vi "Card PXI Information.vi"() -> ()   [LabVIEW 2019]
doc: "This example reports the card PXI signal information, displays the current state\nof the various PXI discrete I/O pins, is capable of configuring PXI discrete I/Os as \noutput using the \"Enable\" toggle, Assert or Deassert output-enabled signals using \nthe \"Drive\" toggle and is capable of sourcing the 10MHz timing signal on the \nDSTARC line."
uses:
  <instrlib>/BTICardLib/Public/Controls/PXI Signal.ctl
  <instrlib>/BTICardLib/Private/Initialize By Card Number and Core Number.vi
  <instrlib>/BTICardLib/BTICardLV.lvlib
panel:
  out "?":bool
  out "?":bool
  out "?":bool
  out "?":bool
  out "?":bool
  out "?":bool
  out "?":bool
  out "?":bool
  out "?":bool
  out "?":bool
  out "?":bool
  in  "?":bool
  in  "?":bool
  in  "?":bool
  in  "?":bool
  in  "?":bool
  in  "?":bool
  in  "?":bool
  in  "?":bool
  in  "?":bool
  in  "?":bool
  in  "?":bool
  in  "?":bool
  in  "?":bool
  in  "?":bool
  in  "?":bool
  in  "?":bool
  in  "?":bool
  in  "?":bool
  in  "?":bool
  in  "?":bool
  in  "?":bool
  in  "?":bool
  in  "?":bool
  in  "?":bool
  in  "?":bool
  out "?":bool
  in  "Card Number":i32
  in  "Core Number":i32
  # "Card PXI Information"
  # "©2016 Astronics Ballard Technology"
  # "This example reports the card PXI signal information, displays the current state\nof the various PXI discrete I/O pins, is capable of configuring PXI discrete I/Os as \noutput using the \"Enable\" toggle, Assert or Deassert output-enabled signals using \nthe \"Drive\" toggle and is capable of sourcing the 10MHz timing signal on the \nDSTARC line."
  # "Signal High/Low"
  # "Enable"
  # "Drive"
  # "PXI_TRIG0"
  # "PXI_TRIG1"
  # "PXI_TRIG2"
  # "PXI_TRIG3"
  # "PXI_TRIG4"
  # "PXI_TRIG5"
  # "PXI_TRIG6"
  # "PXI_TRIG7"
  # "PXIE_DSTARA"
  # "PXIE_DSTARB"
  # "PXI_STAR"
  # "PXIE_DSTARC"
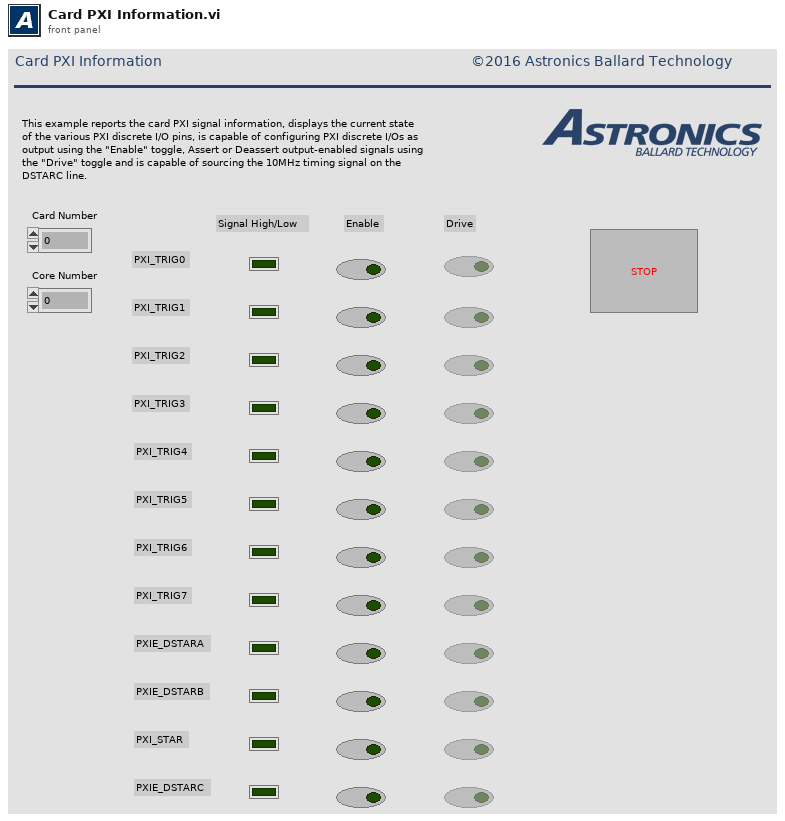
[diagram p1: front panel]
types:
  T1 = enum8{"Enabled", "Disabled", "Disabled and Grayed Out"}
  T2 = typedef "BTICardLV.lvlib/PXI Signal.ctl" = u32
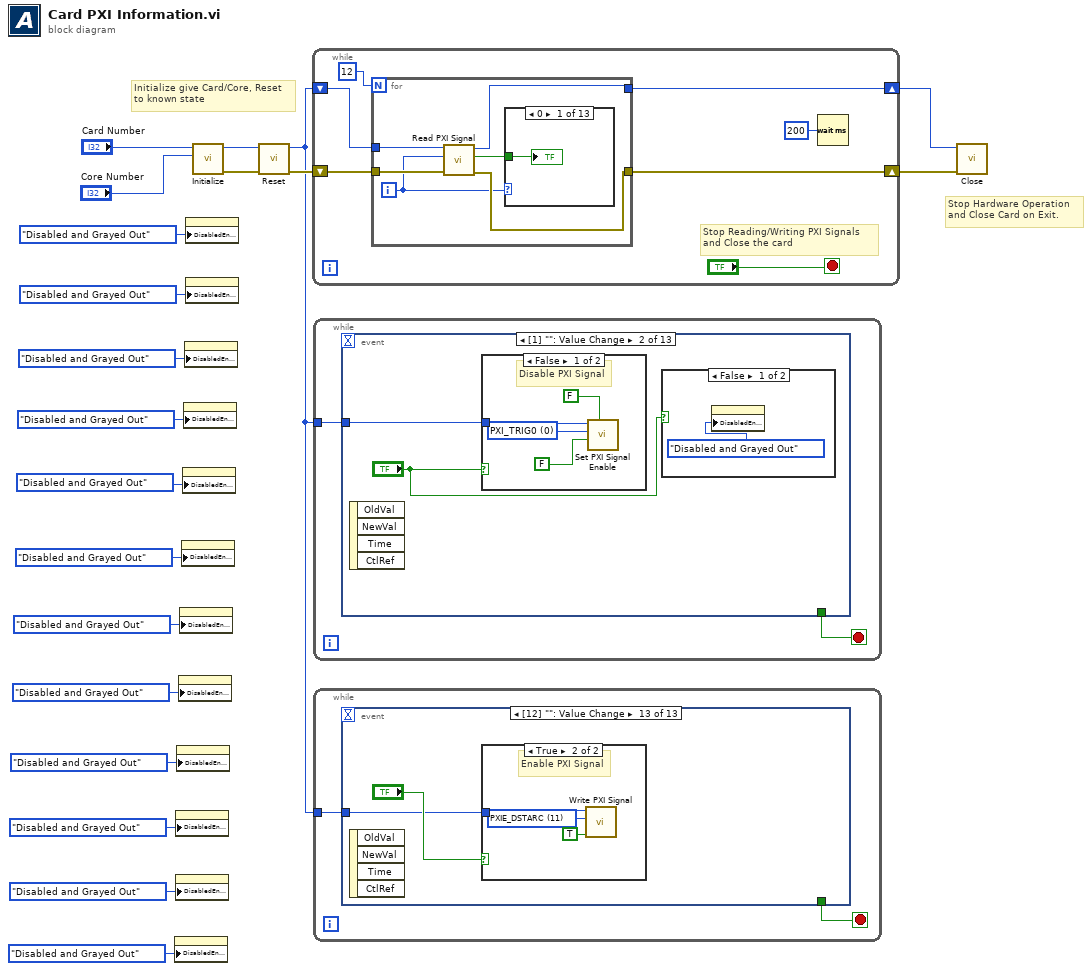
[diagram p0: block diagram]
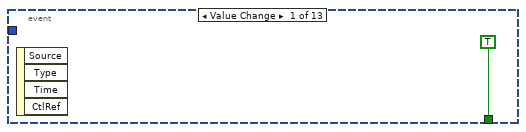
[diagram p2: hidden frame]
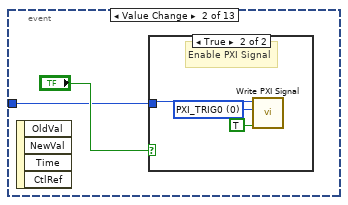
[diagram p3: hidden frame]
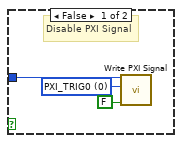
[diagram p4: hidden frame]
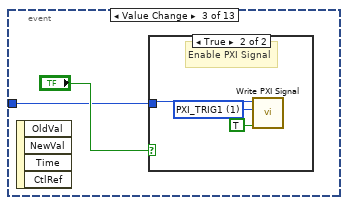
[diagram p5: hidden frame]
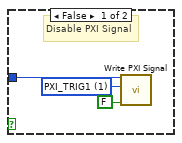
[diagram p6: hidden frame]
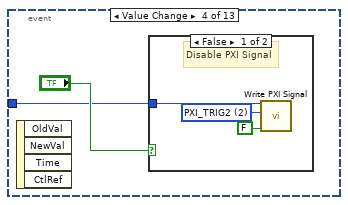
[diagram p7: hidden frame]
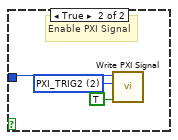
[diagram p8: hidden frame]
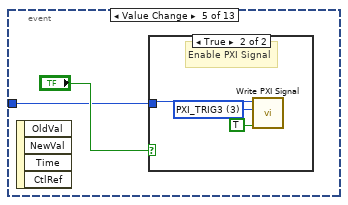
[diagram p9: hidden frame]
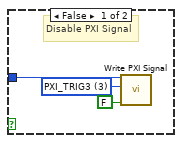
[diagram p10: hidden frame]
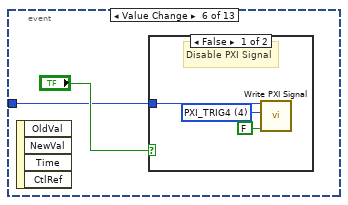
[diagram p11: hidden frame]
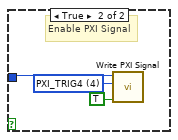
[diagram p12: hidden frame]
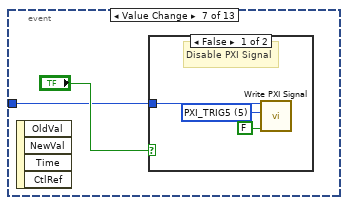
[diagram p13: hidden frame]
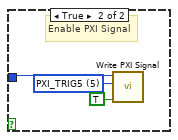
[diagram p14: hidden frame]
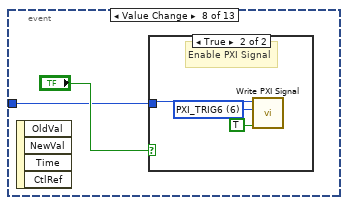
[diagram p15: hidden frame]
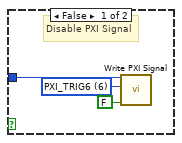
[diagram p16: hidden frame]
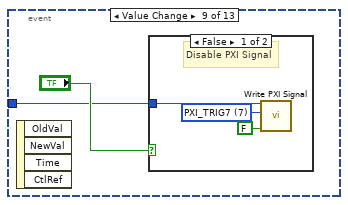
[diagram p17: hidden frame]
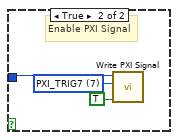
[diagram p18: hidden frame]
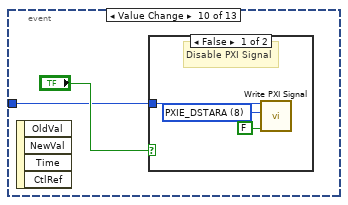
[diagram p19: hidden frame]
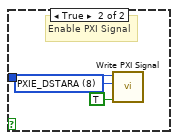
[diagram p20: hidden frame]
diagram:
  # "Stop Hardware Operation\nand Close Card on Exit."
  # "Initialize give Card/Core, Reset\nto known state"
  n1 = property class="Bool (strict)"("DisabledEnum"=T1."Disabled and Grayed Out" ("Disabled")) -> ()  [unwired: 2 in, 2 out]
  n2 = property class="Bool (strict)"("DisabledEnum"=T1."Disabled and Grayed Out" ("Disabled")) -> ()  [unwired: 2 in, 2 out]
  n3 = property class="Bool (strict)"("DisabledEnum"=T1."Disabled and Grayed Out" ("Disabled")) -> ()  [unwired: 2 in, 2 out]
  n4 = property class="Bool (strict)"("DisabledEnum"=T1."Disabled and Grayed Out" ("Disabled")) -> ()  [unwired: 2 in, 2 out]
  n5 = property class="Bool (strict)"("DisabledEnum"=T1."Disabled and Grayed Out" ("Disabled")) -> ()  [unwired: 2 in, 2 out]
  n6 = property class="Bool (strict)"("DisabledEnum"=T1."Disabled and Grayed Out" ("Disabled")) -> ()  [unwired: 2 in, 2 out]
  n7 = property class="Bool (strict)"("DisabledEnum"=T1."Disabled and Grayed Out" ("Disabled")) -> ()  [unwired: 2 in, 2 out]
  n8 = property class="Bool (strict)"("DisabledEnum"=T1."Disabled and Grayed Out" ("Disabled")) -> ()  [unwired: 2 in, 2 out]
  n9 = property class="Bool (strict)"("DisabledEnum"=T1."Disabled and Grayed Out" ("Disabled")) -> ()  [unwired: 2 in, 2 out]
  n10 = property class="Bool (strict)"("DisabledEnum"=T1."Disabled and Grayed Out" ("Disabled")) -> ()  [unwired: 2 in, 2 out]
  n11 = property class="Bool (strict)"("DisabledEnum"=T1."Disabled and Grayed Out" ("Disabled")) -> ()  [unwired: 2 in, 2 out]
  n12 = property class="Bool (strict)"("DisabledEnum"=T1."Disabled and Grayed Out" ("Disabled")) -> ()  [unwired: 2 in, 2 out]
  n13 = call-poly <instrlib>:"Initialize.vi"("core number"="Core Number", "card number"="Card Number") -> ("error out"=w17:errorcluster, "core handle out"=w18:u64)  [unwired: 8 in]
  n14 = call <instrlib>:"Reset.vi"("error in (no error)"=w17, "core handle in"=w18) -> ("error out"=w16:errorcluster, "core handle out"=w13:u64)  [unwired: 8 in]
  n15 = while {
    shift-right: [w23] -> w14
    shift-left: w13 -> [w26]
    shift-right: [w24] -> w15
    shift-left: w16 -> [w25]
    stop <- "?" stop-if-true
    # "Stop Reading/Writing PXI Signals\nand Close the card"
    n16 = for {
      N: 12 -> [_]
      tunnel: w26 -> [w33]
      tunnel: w25 -> [w32]
      tunnel: [w31] -> w24
      tunnel: [w30] -> w23
      i -> [w29]
      n17 = call <instrlib>:"Read PXI Signal.vi"("error in (no error)"=w32, "pxi signal"=w29, "core handle in"=w33) -> ("error out"=w31:errorcluster, "signal value"=w28:bool, "core handle out"=w30:u64)  [unwired: 6 in]
      n18 = case shown="0" w29 {
        tunnel: w28 -> [w34 w35 w36 w37 w38 w39 w40 w41 w42 w43 w44 w45 _]
        frame 0 {
          "?" <- w34
        }
        frame 1 {
          "?" <- w35
        }
        frame 2 {
          "?" <- w36
        }
        frame 3 {
          "?" <- w37
        }
        frame 4 {
          "?" <- w38
        }
        frame 5 {
          "?" <- w39
        }
        frame 6 {
          "?" <- w40
        }
        frame 7 {
          "?" <- w41
        }
        frame 8 {
          "?" <- w42
        }
        frame 9 {
          "?" <- w43
        }
        frame 10 {
          "?" <- w44
        }
        frame 11 {
          "?" <- w45
        }
        frame 12, Default {
        }
      }
    }
    n19 = Wait (ms)(milliseconds to wait=u32 200) -> ()  [unwired: 1 out]
  }
  n20 = while {
    tunnel: w13 -> [w47]
    stop <- w46 stop-if-true
    n21 = event shown="[1] \"\": Value Change" {
      selector: _ -> [_ _ _ _ _ _ _ _ _ _ _ _ _]
      dyn-events: _ -> [_ _ _ _ _ _ _ _ _ _ _ _ _]
      timeout: _ -> [_ _ _ _ _ _ _ _ _ _ _ _ _]
      tunnel: w47 -> [_ w49 w61 w73 w85 w97 w109 w121 w133 w145 w157 w169 w181]
      tunnel: [TRUE ("Stop Reading/Writing PXI Signals\nand Close the card") _ _ _ _ _ _ _ _ _ _ _ _] -> w46
      event Value Change {
        n22 = event-data() -> ()  [unwired: 1 in, 4 out]
      }
      event Value Change {
        n23 = event-data() -> ()  [unwired: 1 in, 4 out]
        n24 = case shown="False" "?" {
          tunnel: w49 -> [w54 w60]
          frame False {
            w55 = T2 0 items=["PXI_TRIG0", "PXI_TRIG1", "PXI_TRIG2", "PXI_TRIG3", "PXI_TRIG4", "PXI_TRIG5", "PXI_TRIG6", "PXI_TRIG7", "PXIE_DSTARA", "PXIE_DSTARB", "PXI_STAR", "PXIE_DSTARC"] ("pxi signal")
            # "Disable PXI Signal"
            n25 = call <instrlib>:"Set PXI Signal Enable.vi"("signal value"=FALSE, "output enable?"=FALSE, "pxi signal"=w55, "corehandle in"=w54) -> ()  [unwired: 6 in, 2 out]
          }
          frame True {
            w58 = T2 0 items=["PXI_TRIG0", "PXI_TRIG1", "PXI_TRIG2", "PXI_TRIG3", "PXI_TRIG4", "PXI_TRIG5", "PXI_TRIG6", "PXI_TRIG7", "PXIE_DSTARA", "PXIE_DSTARB", "PXI_STAR", "PXIE_DSTARC"] ("pxi signal")
            # "Enable PXI Signal"
            n26 = call <instrlib>:"Set PXI Signal Enable.vi"("signal value"=FALSE, "output enable?"=TRUE, "pxi signal"=w58, "corehandle in"=w60) -> ()  [unwired: 6 in, 2 out]
          }
        }
        n27 = case shown="False" "?" {
          frame False {
            n28 = property class="Bool (strict)"("DisabledEnum"=T1."Disabled and Grayed Out" ("Disabled")) -> ()  [unwired: 2 in, 2 out]
          }
          frame True {
            n29 = property class="Bool (strict)"("DisabledEnum"=T1."Enabled" ("Disabled")) -> ()  [unwired: 2 in, 2 out]
          }
        }
      }
      event Value Change {
        n30 = event-data() -> ()  [unwired: 1 in, 4 out]
        n31 = case shown="True" "?" {
          tunnel: w61 -> [w66 w72]
          frame False {
            w67 = T2 1 items=["PXI_TRIG0", "PXI_TRIG1", "PXI_TRIG2", "PXI_TRIG3", "PXI_TRIG4", "PXI_TRIG5", "PXI_TRIG6", "PXI_TRIG7", "PXIE_DSTARA", "PXIE_DSTARB", "PXI_STAR", "PXIE_DSTARC"] ("pxi signal")
            # "Disable PXI Signal"
            n32 = call <instrlib>:"Set PXI Signal Enable.vi"("signal value"=FALSE, "output enable?"=FALSE, "pxi signal"=w67, "corehandle in"=w66) -> ()  [unwired: 6 in, 2 out]
          }
          frame True {
            w70 = T2 1 items=["PXI_TRIG0", "PXI_TRIG1", "PXI_TRIG2", "PXI_TRIG3", "PXI_TRIG4", "PXI_TRIG5", "PXI_TRIG6", "PXI_TRIG7", "PXIE_DSTARA", "PXIE_DSTARB", "PXI_STAR", "PXIE_DSTARC"] ("pxi signal")
            # "Enable PXI Signal"
            n33 = call <instrlib>:"Set PXI Signal Enable.vi"("signal value"=FALSE, "output enable?"=TRUE, "pxi signal"=w70, "corehandle in"=w72) -> ()  [unwired: 6 in, 2 out]
          }
        }
        n34 = case shown="True" "?" {
          frame False {
            n35 = property class="Bool (strict)"("DisabledEnum"=T1."Disabled and Grayed Out" ("Disabled")) -> ()  [unwired: 2 in, 2 out]
          }
          frame True {
            n36 = property class="Bool (strict)"("DisabledEnum"=T1."Enabled" ("Disabled")) -> ()  [unwired: 2 in, 2 out]
          }
        }
      }
      event Value Change {
        n37 = event-data() -> ()  [unwired: 1 in, 4 out]
        n38 = case shown="True" "?" {
          tunnel: w73 -> [w78 w84]
          frame False {
            w79 = T2 2 items=["PXI_TRIG0", "PXI_TRIG1", "PXI_TRIG2", "PXI_TRIG3", "PXI_TRIG4", "PXI_TRIG5", "PXI_TRIG6", "PXI_TRIG7", "PXIE_DSTARA", "PXIE_DSTARB", "PXI_STAR", "PXIE_DSTARC"] ("pxi signal")
            # "Disable PXI Signal"
            n39 = call <instrlib>:"Set PXI Signal Enable.vi"("signal value"=FALSE, "output enable?"=FALSE, "pxi signal"=w79, "corehandle in"=w78) -> ()  [unwired: 6 in, 2 out]
          }
          frame True {
            w82 = T2 2 items=["PXI_TRIG0", "PXI_TRIG1", "PXI_TRIG2", "PXI_TRIG3", "PXI_TRIG4", "PXI_TRIG5", "PXI_TRIG6", "PXI_TRIG7", "PXIE_DSTARA", "PXIE_DSTARB", "PXI_STAR", "PXIE_DSTARC"] ("pxi signal")
            # "Enable PXI Signal"
            n40 = call <instrlib>:"Set PXI Signal Enable.vi"("signal value"=FALSE, "output enable?"=TRUE, "pxi signal"=w82, "corehandle in"=w84) -> ()  [unwired: 6 in, 2 out]
          }
        }
        n41 = case shown="True" "?" {
          frame False {
            n42 = property class="Bool (strict)"("DisabledEnum"=T1."Disabled and Grayed Out" ("Disabled")) -> ()  [unwired: 2 in, 2 out]
          }
          frame True {
            n43 = property class="Bool (strict)"("DisabledEnum"=T1."Enabled" ("Disabled")) -> ()  [unwired: 2 in, 2 out]
          }
        }
      }
      event Value Change {
        n44 = event-data() -> ()  [unwired: 1 in, 4 out]
        n45 = case shown="False" "?" {
          tunnel: w85 -> [w90 w96]
          frame False {
            w91 = T2 3 items=["PXI_TRIG0", "PXI_TRIG1", "PXI_TRIG2", "PXI_TRIG3", "PXI_TRIG4", "PXI_TRIG5", "PXI_TRIG6", "PXI_TRIG7", "PXIE_DSTARA", "PXIE_DSTARB", "PXI_STAR", "PXIE_DSTARC"] ("pxi signal")
            # "Disable PXI Signal"
            n46 = call <instrlib>:"Set PXI Signal Enable.vi"("signal value"=FALSE, "output enable?"=FALSE, "pxi signal"=w91, "corehandle in"=w90) -> ()  [unwired: 6 in, 2 out]
          }
          frame True {
            w94 = T2 3 items=["PXI_TRIG0", "PXI_TRIG1", "PXI_TRIG2", "PXI_TRIG3", "PXI_TRIG4", "PXI_TRIG5", "PXI_TRIG6", "PXI_TRIG7", "PXIE_DSTARA", "PXIE_DSTARB", "PXI_STAR", "PXIE_DSTARC"] ("pxi signal")
            # "Enable PXI Signal"
            n47 = call <instrlib>:"Set PXI Signal Enable.vi"("signal value"=FALSE, "output enable?"=TRUE, "pxi signal"=w94, "corehandle in"=w96) -> ()  [unwired: 6 in, 2 out]
          }
        }
        n48 = case shown="False" "?" {
          frame False {
            n49 = property class="Bool (strict)"("DisabledEnum"=T1."Disabled and Grayed Out" ("Disabled")) -> ()  [unwired: 2 in, 2 out]
          }
          frame True {
            n50 = property class="Bool (strict)"("DisabledEnum"=T1."Enabled" ("Disabled")) -> ()  [unwired: 2 in, 2 out]
          }
        }
      }
      event Value Change {
        n51 = event-data() -> ()  [unwired: 1 in, 4 out]
        n52 = case shown="True" "?" {
          tunnel: w97 -> [w102 w108]
          frame False {
            w103 = T2 4 items=["PXI_TRIG0", "PXI_TRIG1", "PXI_TRIG2", "PXI_TRIG3", "PXI_TRIG4", "PXI_TRIG5", "PXI_TRIG6", "PXI_TRIG7", "PXIE_DSTARA", "PXIE_DSTARB", "PXI_STAR", "PXIE_DSTARC"] ("pxi signal")
            # "Disable PXI Signal"
            n53 = call <instrlib>:"Set PXI Signal Enable.vi"("signal value"=FALSE, "output enable?"=FALSE, "pxi signal"=w103, "corehandle in"=w102) -> ()  [unwired: 6 in, 2 out]
          }
          frame True {
            w106 = T2 4 items=["PXI_TRIG0", "PXI_TRIG1", "PXI_TRIG2", "PXI_TRIG3", "PXI_TRIG4", "PXI_TRIG5", "PXI_TRIG6", "PXI_TRIG7", "PXIE_DSTARA", "PXIE_DSTARB", "PXI_STAR", "PXIE_DSTARC"] ("pxi signal")
            # "Enable PXI Signal"
            n54 = call <instrlib>:"Set PXI Signal Enable.vi"("signal value"=FALSE, "output enable?"=TRUE, "pxi signal"=w106, "corehandle in"=w108) -> ()  [unwired: 6 in, 2 out]
          }
        }
        n55 = case shown="True" "?" {
          frame False {
            n56 = property class="Bool (strict)"("DisabledEnum"=T1."Disabled and Grayed Out" ("Disabled")) -> ()  [unwired: 2 in, 2 out]
          }
          frame True {
            n57 = property class="Bool (strict)"("DisabledEnum"=T1."Enabled" ("Disabled")) -> ()  [unwired: 2 in, 2 out]
          }
        }
      }
      event Value Change {
        n58 = event-data() -> ()  [unwired: 1 in, 4 out]
        n59 = case shown="True" "?" {
          tunnel: w109 -> [w114 w120]
          frame False {
            w115 = T2 5 items=["PXI_TRIG0", "PXI_TRIG1", "PXI_TRIG2", "PXI_TRIG3", "PXI_TRIG4", "PXI_TRIG5", "PXI_TRIG6", "PXI_TRIG7", "PXIE_DSTARA", "PXIE_DSTARB", "PXI_STAR", "PXIE_DSTARC"] ("pxi signal")
            # "Disable PXI Signal"
            n60 = call <instrlib>:"Set PXI Signal Enable.vi"("signal value"=FALSE, "output enable?"=FALSE, "pxi signal"=w115, "corehandle in"=w114) -> ()  [unwired: 6 in, 2 out]
          }
          frame True {
            w118 = T2 5 items=["PXI_TRIG0", "PXI_TRIG1", "PXI_TRIG2", "PXI_TRIG3", "PXI_TRIG4", "PXI_TRIG5", "PXI_TRIG6", "PXI_TRIG7", "PXIE_DSTARA", "PXIE_DSTARB", "PXI_STAR", "PXIE_DSTARC"] ("pxi signal")
            # "Enable PXI Signal"
            n61 = call <instrlib>:"Set PXI Signal Enable.vi"("signal value"=FALSE, "output enable?"=TRUE, "pxi signal"=w118, "corehandle in"=w120) -> ()  [unwired: 6 in, 2 out]
          }
        }
        n62 = case shown="True" "?" {
          frame False {
            n63 = property class="Bool (strict)"("DisabledEnum"=T1."Disabled and Grayed Out" ("Disabled")) -> ()  [unwired: 2 in, 2 out]
          }
          frame True {
            n64 = property class="Bool (strict)"("DisabledEnum"=T1."Enabled" ("Disabled")) -> ()  [unwired: 2 in, 2 out]
          }
        }
      }
      event Value Change {
        n65 = event-data() -> ()  [unwired: 1 in, 4 out]
        n66 = case shown="False" "?" {
          tunnel: w121 -> [w126 w132]
          frame False {
            w127 = T2 6 items=["PXI_TRIG0", "PXI_TRIG1", "PXI_TRIG2", "PXI_TRIG3", "PXI_TRIG4", "PXI_TRIG5", "PXI_TRIG6", "PXI_TRIG7", "PXIE_DSTARA", "PXIE_DSTARB", "PXI_STAR", "PXIE_DSTARC"] ("pxi signal")
            # "Disable PXI Signal"
            n67 = call <instrlib>:"Set PXI Signal Enable.vi"("signal value"=FALSE, "output enable?"=FALSE, "pxi signal"=w127, "corehandle in"=w126) -> ()  [unwired: 6 in, 2 out]
          }
          frame True {
            w130 = T2 6 items=["PXI_TRIG0", "PXI_TRIG1", "PXI_TRIG2", "PXI_TRIG3", "PXI_TRIG4", "PXI_TRIG5", "PXI_TRIG6", "PXI_TRIG7", "PXIE_DSTARA", "PXIE_DSTARB", "PXI_STAR", "PXIE_DSTARC"] ("pxi signal")
            # "Enable PXI Signal"
            n68 = call <instrlib>:"Set PXI Signal Enable.vi"("signal value"=FALSE, "output enable?"=TRUE, "pxi signal"=w130, "corehandle in"=w132) -> ()  [unwired: 6 in, 2 out]
          }
        }
        n69 = case shown="True" "?" {
          frame False {
            n70 = property class="Bool (strict)"("DisabledEnum"=T1."Disabled and Grayed Out" ("Disabled")) -> ()  [unwired: 2 in, 2 out]
          }
          frame True {
            n71 = property class="Bool (strict)"("DisabledEnum"=T1."Enabled" ("Disabled")) -> ()  [unwired: 2 in, 2 out]
          }
        }
      }
      event Value Change {
        n72 = event-data() -> ()  [unwired: 1 in, 4 out]
        n73 = case shown="True" "?" {
          tunnel: w133 -> [w138 w144]
          frame False {
            w139 = T2 7 items=["PXI_TRIG0", "PXI_TRIG1", "PXI_TRIG2", "PXI_TRIG3", "PXI_TRIG4", "PXI_TRIG5", "PXI_TRIG6", "PXI_TRIG7", "PXIE_DSTARA", "PXIE_DSTARB", "PXI_STAR", "PXIE_DSTARC"] ("pxi signal")
            # "Disable PXI Signal"
            n74 = call <instrlib>:"Set PXI Signal Enable.vi"("signal value"=FALSE, "output enable?"=FALSE, "pxi signal"=w139, "corehandle in"=w138) -> ()  [unwired: 6 in, 2 out]
          }
          frame True {
            w142 = T2 7 items=["PXI_TRIG0", "PXI_TRIG1", "PXI_TRIG2", "PXI_TRIG3", "PXI_TRIG4", "PXI_TRIG5", "PXI_TRIG6", "PXI_TRIG7", "PXIE_DSTARA", "PXIE_DSTARB", "PXI_STAR", "PXIE_DSTARC"] ("pxi signal")
            # "Enable PXI Signal"
            n75 = call <instrlib>:"Set PXI Signal Enable.vi"("signal value"=FALSE, "output enable?"=TRUE, "pxi signal"=w142, "corehandle in"=w144) -> ()  [unwired: 6 in, 2 out]
          }
        }
        n76 = case shown="False" "?" {
          frame False {
            n77 = property class="Bool (strict)"("DisabledEnum"=T1."Disabled and Grayed Out" ("Disabled")) -> ()  [unwired: 2 in, 2 out]
          }
          frame True {
            n78 = property class="Bool (strict)"("DisabledEnum"=T1."Enabled" ("Disabled")) -> ()  [unwired: 2 in, 2 out]
          }
        }
      }
      event Value Change {
        n79 = event-data() -> ()  [unwired: 1 in, 4 out]
        n80 = case shown="True" "?" {
          tunnel: w145 -> [w150 w156]
          frame False {
            w151 = T2 8 items=["PXI_TRIG0", "PXI_TRIG1", "PXI_TRIG2", "PXI_TRIG3", "PXI_TRIG4", "PXI_TRIG5", "PXI_TRIG6", "PXI_TRIG7", "PXIE_DSTARA", "PXIE_DSTARB", "PXI_STAR", "PXIE_DSTARC"] ("pxi signal")
            # "Disable PXI Signal"
            n81 = call <instrlib>:"Set PXI Signal Enable.vi"("signal value"=FALSE, "output enable?"=FALSE, "pxi signal"=w151, "corehandle in"=w150) -> ()  [unwired: 6 in, 2 out]
          }
          frame True {
            w154 = T2 8 items=["PXI_TRIG0", "PXI_TRIG1", "PXI_TRIG2", "PXI_TRIG3", "PXI_TRIG4", "PXI_TRIG5", "PXI_TRIG6", "PXI_TRIG7", "PXIE_DSTARA", "PXIE_DSTARB", "PXI_STAR", "PXIE_DSTARC"] ("pxi signal")
            # "Enable PXI Signal"
            n82 = call <instrlib>:"Set PXI Signal Enable.vi"("signal value"=FALSE, "output enable?"=TRUE, "pxi signal"=w154, "corehandle in"=w156) -> ()  [unwired: 6 in, 2 out]
          }
        }
        n83 = case shown="True" "?" {
          frame False {
            n84 = property class="Bool (strict)"("DisabledEnum"=T1."Disabled and Grayed Out" ("Disabled")) -> ()  [unwired: 2 in, 2 out]
          }
          frame True {
            n85 = property class="Bool (strict)"("DisabledEnum"=T1."Enabled" ("Disabled")) -> ()  [unwired: 2 in, 2 out]
          }
        }
      }
      event Value Change {
        n86 = event-data() -> ()  [unwired: 1 in, 4 out]
        n87 = case shown="True" "?" {
          tunnel: w157 -> [w162 w168]
          frame False {
            w163 = T2 9 items=["PXI_TRIG0", "PXI_TRIG1", "PXI_TRIG2", "PXI_TRIG3", "PXI_TRIG4", "PXI_TRIG5", "PXI_TRIG6", "PXI_TRIG7", "PXIE_DSTARA", "PXIE_DSTARB", "PXI_STAR", "PXIE_DSTARC"] ("pxi signal")
            # "Disable PXI Signal"
            n88 = call <instrlib>:"Set PXI Signal Enable.vi"("signal value"=FALSE, "output enable?"=FALSE, "pxi signal"=w163, "corehandle in"=w162) -> ()  [unwired: 6 in, 2 out]
          }
          frame True {
            w166 = T2 9 items=["PXI_TRIG0", "PXI_TRIG1", "PXI_TRIG2", "PXI_TRIG3", "PXI_TRIG4", "PXI_TRIG5", "PXI_TRIG6", "PXI_TRIG7", "PXIE_DSTARA", "PXIE_DSTARB", "PXI_STAR", "PXIE_DSTARC"] ("pxi signal")
            # "Enable PXI Signal"
            n89 = call <instrlib>:"Set PXI Signal Enable.vi"("signal value"=FALSE, "output enable?"=TRUE, "pxi signal"=w166, "corehandle in"=w168) -> ()  [unwired: 6 in, 2 out]
          }
        }
        n90 = case shown="True" "?" {
          frame False {
            n91 = property class="Bool (strict)"("DisabledEnum"=T1."Disabled and Grayed Out" ("Disabled")) -> ()  [unwired: 2 in, 2 out]
          }
          frame True {
            n92 = property class="Bool (strict)"("DisabledEnum"=T1."Enabled" ("Disabled")) -> ()  [unwired: 2 in, 2 out]
          }
        }
      }
      event Value Change {
        n93 = event-data() -> ()  [unwired: 1 in, 4 out]
        n94 = case shown="False" "?" {
          tunnel: w169 -> [w174 w180]
          frame False {
            w175 = T2 10 items=["PXI_TRIG0", "PXI_TRIG1", "PXI_TRIG2", "PXI_TRIG3", "PXI_TRIG4", "PXI_TRIG5", "PXI_TRIG6", "PXI_TRIG7", "PXIE_DSTARA", "PXIE_DSTARB", "PXI_STAR", "PXIE_DSTARC"] ("pxi signal")
            # "Disable PXI Signal"
            n95 = call <instrlib>:"Set PXI Signal Enable.vi"("signal value"=FALSE, "output enable?"=FALSE, "pxi signal"=w175, "corehandle in"=w174) -> ()  [unwired: 6 in, 2 out]
          }
          frame True {
            w178 = T2 10 items=["PXI_TRIG0", "PXI_TRIG1", "PXI_TRIG2", "PXI_TRIG3", "PXI_TRIG4", "PXI_TRIG5", "PXI_TRIG6", "PXI_TRIG7", "PXIE_DSTARA", "PXIE_DSTARB", "PXI_STAR", "PXIE_DSTARC"] ("pxi signal")
            # "Enable PXI Signal"
            n96 = call <instrlib>:"Set PXI Signal Enable.vi"("signal value"=FALSE, "output enable?"=TRUE, "pxi signal"=w178, "corehandle in"=w180) -> ()  [unwired: 6 in, 2 out]
          }
        }
        n97 = case shown="True" "?" {
          frame False {
            n98 = property class="Bool (strict)"("DisabledEnum"=T1."Disabled and Grayed Out" ("Disabled")) -> ()  [unwired: 2 in, 2 out]
          }
          frame True {
            n99 = property class="Bool (strict)"("DisabledEnum"=T1."Enabled" ("Disabled")) -> ()  [unwired: 2 in, 2 out]
          }
        }
      }
      event Value Change {
        n100 = event-data() -> ()  [unwired: 1 in, 4 out]
        n101 = case shown="True" "?" {
          tunnel: w181 -> [w186 w192]
          frame False {
            w187 = T2 11 items=["PXI_TRIG0", "PXI_TRIG1", "PXI_TRIG2", "PXI_TRIG3", "PXI_TRIG4", "PXI_TRIG5", "PXI_TRIG6", "PXI_TRIG7", "PXIE_DSTARA", "PXIE_DSTARB", "PXI_STAR", "PXIE_DSTARC"] ("pxi signal")
            # "Disable PXI Signal"
            n102 = call <instrlib>:"Set PXI Signal Enable.vi"("signal value"=FALSE, "output enable?"=FALSE, "pxi signal"=w187, "corehandle in"=w186) -> ()  [unwired: 6 in, 2 out]
          }
          frame True {
            w190 = T2 11 items=["PXI_TRIG0", "PXI_TRIG1", "PXI_TRIG2", "PXI_TRIG3", "PXI_TRIG4", "PXI_TRIG5", "PXI_TRIG6", "PXI_TRIG7", "PXIE_DSTARA", "PXIE_DSTARB", "PXI_STAR", "PXIE_DSTARC"] ("pxi signal")
            # "Enable PXI Signal"
            n103 = call <instrlib>:"Set PXI Signal Enable.vi"("signal value"=FALSE, "output enable?"=TRUE, "pxi signal"=w190, "corehandle in"=w192) -> ()  [unwired: 6 in, 2 out]
          }
        }
        n104 = case shown="True" "?" {
          frame False {
            n105 = property class="Bool (strict)"("DisabledEnum"=T1."Disabled and Grayed Out" ("Disabled")) -> ()  [unwired: 2 in, 2 out]
          }
          frame True {
            n106 = property class="Bool (strict)"("DisabledEnum"=T1."Enabled" ("Disabled")) -> ()  [unwired: 2 in, 2 out]
          }
        }
      }
    }
  }
  n107 = while {
    tunnel: w13 -> [w193]
    stop <- w194 stop-if-true
    n108 = event shown="[12] \"\": Value Change" {
      selector: _ -> [_ _ _ _ _ _ _ _ _ _ _ _ _]
      dyn-events: _ -> [_ _ _ _ _ _ _ _ _ _ _ _ _]
      timeout: _ -> [_ _ _ _ _ _ _ _ _ _ _ _ _]
      tunnel: [TRUE ("Stop Reading/Writing PXI Signals\nand Close the card") _ _ _ _ _ _ _ _ _ _ _ _] -> w194
      tunnel: w193 -> [_ w196 w204 w212 w220 w228 w236 w244 w252 w260 w268 w276 w284]
      event Value Change {
        n109 = event-data() -> ()  [unwired: 1 in, 4 out]
      }
      event Value Change {
        n110 = event-data() -> ()  [unwired: 1 in, 4 out]
        n111 = case shown="True" "?" {
          tunnel: w196 -> [w198 w203]
          frame False {
            w200 = T2 0 items=["PXI_TRIG0", "PXI_TRIG1", "PXI_TRIG2", "PXI_TRIG3", "PXI_TRIG4", "PXI_TRIG5", "PXI_TRIG6", "PXI_TRIG7", "PXIE_DSTARA", "PXIE_DSTARB", "PXI_STAR", "PXIE_DSTARC"] ("pxi signal")
            # "Disable PXI Signal"
            n112 = call <instrlib>:"Write PXI Signal.vi"("signal value"=FALSE, "pxi signal"=w200, "core handle in"=w198) -> ()  [unwired: 7 in, 2 out]
          }
          frame True {
            w202 = T2 0 items=["PXI_TRIG0", "PXI_TRIG1", "PXI_TRIG2", "PXI_TRIG3", "PXI_TRIG4", "PXI_TRIG5", "PXI_TRIG6", "PXI_TRIG7", "PXIE_DSTARA", "PXIE_DSTARB", "PXI_STAR", "PXIE_DSTARC"] ("pxi signal")
            # "Enable PXI Signal"
            n113 = call <instrlib>:"Write PXI Signal.vi"("signal value"=TRUE, "pxi signal"=w202, "core handle in"=w203) -> ()  [unwired: 7 in, 2 out]
          }
        }
      }
      event Value Change {
        n114 = event-data() -> ()  [unwired: 1 in, 4 out]
        n115 = case shown="True" "?" {
          tunnel: w204 -> [w206 w211]
          frame False {
            w208 = T2 1 items=["PXI_TRIG0", "PXI_TRIG1", "PXI_TRIG2", "PXI_TRIG3", "PXI_TRIG4", "PXI_TRIG5", "PXI_TRIG6", "PXI_TRIG7", "PXIE_DSTARA", "PXIE_DSTARB", "PXI_STAR", "PXIE_DSTARC"] ("pxi signal")
            # "Disable PXI Signal"
            n116 = call <instrlib>:"Write PXI Signal.vi"("signal value"=FALSE, "pxi signal"=w208, "core handle in"=w206) -> ()  [unwired: 7 in, 2 out]
          }
          frame True {
            w210 = T2 1 items=["PXI_TRIG0", "PXI_TRIG1", "PXI_TRIG2", "PXI_TRIG3", "PXI_TRIG4", "PXI_TRIG5", "PXI_TRIG6", "PXI_TRIG7", "PXIE_DSTARA", "PXIE_DSTARB", "PXI_STAR", "PXIE_DSTARC"] ("pxi signal")
            # "Enable PXI Signal"
            n117 = call <instrlib>:"Write PXI Signal.vi"("signal value"=TRUE, "pxi signal"=w210, "core handle in"=w211) -> ()  [unwired: 7 in, 2 out]
          }
        }
      }
      event Value Change {
        n118 = event-data() -> ()  [unwired: 1 in, 4 out]
        n119 = case shown="False" "?" {
          tunnel: w212 -> [w214 w219]
          frame False {
            w216 = T2 2 items=["PXI_TRIG0", "PXI_TRIG1", "PXI_TRIG2", "PXI_TRIG3", "PXI_TRIG4", "PXI_TRIG5", "PXI_TRIG6", "PXI_TRIG7", "PXIE_DSTARA", "PXIE_DSTARB", "PXI_STAR", "PXIE_DSTARC"] ("pxi signal")
            # "Disable PXI Signal"
            n120 = call <instrlib>:"Write PXI Signal.vi"("signal value"=FALSE, "pxi signal"=w216, "core handle in"=w214) -> ()  [unwired: 7 in, 2 out]
          }
          frame True {
            w218 = T2 2 items=["PXI_TRIG0", "PXI_TRIG1", "PXI_TRIG2", "PXI_TRIG3", "PXI_TRIG4", "PXI_TRIG5", "PXI_TRIG6", "PXI_TRIG7", "PXIE_DSTARA", "PXIE_DSTARB", "PXI_STAR", "PXIE_DSTARC"] ("pxi signal")
            # "Enable PXI Signal"
            n121 = call <instrlib>:"Write PXI Signal.vi"("signal value"=TRUE, "pxi signal"=w218, "core handle in"=w219) -> ()  [unwired: 7 in, 2 out]
          }
        }
      }
      event Value Change {
        n122 = event-data() -> ()  [unwired: 1 in, 4 out]
        n123 = case shown="True" "?" {
          tunnel: w220 -> [w222 w227]
          frame False {
            w224 = T2 3 items=["PXI_TRIG0", "PXI_TRIG1", "PXI_TRIG2", "PXI_TRIG3", "PXI_TRIG4", "PXI_TRIG5", "PXI_TRIG6", "PXI_TRIG7", "PXIE_DSTARA", "PXIE_DSTARB", "PXI_STAR", "PXIE_DSTARC"] ("pxi signal")
            # "Disable PXI Signal"
            n124 = call <instrlib>:"Write PXI Signal.vi"("signal value"=FALSE, "pxi signal"=w224, "core handle in"=w222) -> ()  [unwired: 7 in, 2 out]
          }
          frame True {
            w226 = T2 3 items=["PXI_TRIG0", "PXI_TRIG1", "PXI_TRIG2", "PXI_TRIG3", "PXI_TRIG4", "PXI_TRIG5", "PXI_TRIG6", "PXI_TRIG7", "PXIE_DSTARA", "PXIE_DSTARB", "PXI_STAR", "PXIE_DSTARC"] ("pxi signal")
            # "Enable PXI Signal"
            n125 = call <instrlib>:"Write PXI Signal.vi"("signal value"=TRUE, "pxi signal"=w226, "core handle in"=w227) -> ()  [unwired: 7 in, 2 out]
          }
        }
      }
      event Value Change {
        n126 = event-data() -> ()  [unwired: 1 in, 4 out]
        n127 = case shown="False" "?" {
          tunnel: w228 -> [w230 w235]
          frame False {
            w232 = T2 4 items=["PXI_TRIG0", "PXI_TRIG1", "PXI_TRIG2", "PXI_TRIG3", "PXI_TRIG4", "PXI_TRIG5", "PXI_TRIG6", "PXI_TRIG7", "PXIE_DSTARA", "PXIE_DSTARB", "PXI_STAR", "PXIE_DSTARC"] ("pxi signal")
            # "Disable PXI Signal"
            n128 = call <instrlib>:"Write PXI Signal.vi"("signal value"=FALSE, "pxi signal"=w232, "core handle in"=w230) -> ()  [unwired: 7 in, 2 out]
          }
          frame True {
            w234 = T2 4 items=["PXI_TRIG0", "PXI_TRIG1", "PXI_TRIG2", "PXI_TRIG3", "PXI_TRIG4", "PXI_TRIG5", "PXI_TRIG6", "PXI_TRIG7", "PXIE_DSTARA", "PXIE_DSTARB", "PXI_STAR", "PXIE_DSTARC"] ("pxi signal")
            # "Enable PXI Signal"
            n129 = call <instrlib>:"Write PXI Signal.vi"("signal value"=TRUE, "pxi signal"=w234, "core handle in"=w235) -> ()  [unwired: 7 in, 2 out]
          }
        }
      }
      event Value Change {
        n130 = event-data() -> ()  [unwired: 1 in, 4 out]
        n131 = case shown="False" "?" {
          tunnel: w236 -> [w238 w243]
          frame False {
            w240 = T2 5 items=["PXI_TRIG0", "PXI_TRIG1", "PXI_TRIG2", "PXI_TRIG3", "PXI_TRIG4", "PXI_TRIG5", "PXI_TRIG6", "PXI_TRIG7", "PXIE_DSTARA", "PXIE_DSTARB", "PXI_STAR", "PXIE_DSTARC"] ("pxi signal")
            # "Disable PXI Signal"
            n132 = call <instrlib>:"Write PXI Signal.vi"("signal value"=FALSE, "pxi signal"=w240, "core handle in"=w238) -> ()  [unwired: 7 in, 2 out]
          }
          frame True {
            w242 = T2 5 items=["PXI_TRIG0", "PXI_TRIG1", "PXI_TRIG2", "PXI_TRIG3", "PXI_TRIG4", "PXI_TRIG5", "PXI_TRIG6", "PXI_TRIG7", "PXIE_DSTARA", "PXIE_DSTARB", "PXI_STAR", "PXIE_DSTARC"] ("pxi signal")
            # "Enable PXI Signal"
            n133 = call <instrlib>:"Write PXI Signal.vi"("signal value"=TRUE, "pxi signal"=w242, "core handle in"=w243) -> ()  [unwired: 7 in, 2 out]
          }
        }
      }
      event Value Change {
        n134 = event-data() -> ()  [unwired: 1 in, 4 out]
        n135 = case shown="True" "?" {
          tunnel: w244 -> [w246 w251]
          frame False {
            w248 = T2 6 items=["PXI_TRIG0", "PXI_TRIG1", "PXI_TRIG2", "PXI_TRIG3", "PXI_TRIG4", "PXI_TRIG5", "PXI_TRIG6", "PXI_TRIG7", "PXIE_DSTARA", "PXIE_DSTARB", "PXI_STAR", "PXIE_DSTARC"] ("pxi signal")
            # "Disable PXI Signal"
            n136 = call <instrlib>:"Write PXI Signal.vi"("signal value"=FALSE, "pxi signal"=w248, "core handle in"=w246) -> ()  [unwired: 7 in, 2 out]
          }
          frame True {
            w250 = T2 6 items=["PXI_TRIG0", "PXI_TRIG1", "PXI_TRIG2", "PXI_TRIG3", "PXI_TRIG4", "PXI_TRIG5", "PXI_TRIG6", "PXI_TRIG7", "PXIE_DSTARA", "PXIE_DSTARB", "PXI_STAR", "PXIE_DSTARC"] ("pxi signal")
            # "Enable PXI Signal"
            n137 = call <instrlib>:"Write PXI Signal.vi"("signal value"=TRUE, "pxi signal"=w250, "core handle in"=w251) -> ()  [unwired: 7 in, 2 out]
          }
        }
      }
      event Value Change {
        n138 = event-data() -> ()  [unwired: 1 in, 4 out]
        n139 = case shown="False" "?" {
          tunnel: w252 -> [w254 w259]
          frame False {
            w256 = T2 7 items=["PXI_TRIG0", "PXI_TRIG1", "PXI_TRIG2", "PXI_TRIG3", "PXI_TRIG4", "PXI_TRIG5", "PXI_TRIG6", "PXI_TRIG7", "PXIE_DSTARA", "PXIE_DSTARB", "PXI_STAR", "PXIE_DSTARC"] ("pxi signal")
            # "Disable PXI Signal"
            n140 = call <instrlib>:"Write PXI Signal.vi"("signal value"=FALSE, "pxi signal"=w256, "core handle in"=w254) -> ()  [unwired: 7 in, 2 out]
          }
          frame True {
            w258 = T2 7 items=["PXI_TRIG0", "PXI_TRIG1", "PXI_TRIG2", "PXI_TRIG3", "PXI_TRIG4", "PXI_TRIG5", "PXI_TRIG6", "PXI_TRIG7", "PXIE_DSTARA", "PXIE_DSTARB", "PXI_STAR", "PXIE_DSTARC"] ("pxi signal")
            # "Enable PXI Signal"
            n141 = call <instrlib>:"Write PXI Signal.vi"("signal value"=TRUE, "pxi signal"=w258, "core handle in"=w259) -> ()  [unwired: 7 in, 2 out]
          }
        }
      }
      event Value Change {
        n142 = event-data() -> ()  [unwired: 1 in, 4 out]
        n143 = case shown="False" "?" {
          tunnel: w260 -> [w262 w267]
          frame False {
            w264 = T2 8 items=["PXI_TRIG0", "PXI_TRIG1", "PXI_TRIG2", "PXI_TRIG3", "PXI_TRIG4", "PXI_TRIG5", "PXI_TRIG6", "PXI_TRIG7", "PXIE_DSTARA", "PXIE_DSTARB", "PXI_STAR", "PXIE_DSTARC"] ("pxi signal")
            # "Disable PXI Signal"
            n144 = call <instrlib>:"Write PXI Signal.vi"("signal value"=FALSE, "pxi signal"=w264, "core handle in"=w262) -> ()  [unwired: 7 in, 2 out]
          }
          frame True {
            w266 = T2 8 items=["PXI_TRIG0", "PXI_TRIG1", "PXI_TRIG2", "PXI_TRIG3", "PXI_TRIG4", "PXI_TRIG5", "PXI_TRIG6", "PXI_TRIG7", "PXIE_DSTARA", "PXIE_DSTARB", "PXI_STAR", "PXIE_DSTARC"] ("pxi signal")
            # "Enable PXI Signal"
            n145 = call <instrlib>:"Write PXI Signal.vi"("signal value"=TRUE, "pxi signal"=w266, "core handle in"=w267) -> ()  [unwired: 7 in, 2 out]
          }
        }
      }
      event Value Change {
        n146 = event-data() -> ()  [unwired: 1 in, 4 out]
        n147 = case shown="True" "?" {
          tunnel: w268 -> [w270 w275]
          frame False {
            w272 = T2 9 items=["PXI_TRIG0", "PXI_TRIG1", "PXI_TRIG2", "PXI_TRIG3", "PXI_TRIG4", "PXI_TRIG5", "PXI_TRIG6", "PXI_TRIG7", "PXIE_DSTARA", "PXIE_DSTARB", "PXI_STAR", "PXIE_DSTARC"] ("pxi signal")
            # "Disable PXI Signal"
            n148 = call <instrlib>:"Write PXI Signal.vi"("signal value"=FALSE, "pxi signal"=w272, "core handle in"=w270) -> ()  [unwired: 7 in, 2 out]
          }
          frame True {
            w274 = T2 9 items=["PXI_TRIG0", "PXI_TRIG1", "PXI_TRIG2", "PXI_TRIG3", "PXI_TRIG4", "PXI_TRIG5", "PXI_TRIG6", "PXI_TRIG7", "PXIE_DSTARA", "PXIE_DSTARB", "PXI_STAR", "PXIE_DSTARC"] ("pxi signal")
            # "Enable PXI Signal"
            n149 = call <instrlib>:"Write PXI Signal.vi"("signal value"=TRUE, "pxi signal"=w274, "core handle in"=w275) -> ()  [unwired: 7 in, 2 out]
          }
        }
      }
      event Value Change {
        n150 = event-data() -> ()  [unwired: 1 in, 4 out]
        n151 = case shown="False" "?" {
          tunnel: w276 -> [w278 w283]
          frame False {
            w280 = T2 10 items=["PXI_TRIG0", "PXI_TRIG1", "PXI_TRIG2", "PXI_TRIG3", "PXI_TRIG4", "PXI_TRIG5", "PXI_TRIG6", "PXI_TRIG7", "PXIE_DSTARA", "PXIE_DSTARB", "PXI_STAR", "PXIE_DSTARC"] ("pxi signal")
            # "Disable PXI Signal"
            n152 = call <instrlib>:"Write PXI Signal.vi"("signal value"=FALSE, "pxi signal"=w280, "core handle in"=w278) -> ()  [unwired: 7 in, 2 out]
          }
          frame True {
            w282 = T2 10 items=["PXI_TRIG0", "PXI_TRIG1", "PXI_TRIG2", "PXI_TRIG3", "PXI_TRIG4", "PXI_TRIG5", "PXI_TRIG6", "PXI_TRIG7", "PXIE_DSTARA", "PXIE_DSTARB", "PXI_STAR", "PXIE_DSTARC"] ("pxi signal")
            # "Enable PXI Signal"
            n153 = call <instrlib>:"Write PXI Signal.vi"("signal value"=TRUE, "pxi signal"=w282, "core handle in"=w283) -> ()  [unwired: 7 in, 2 out]
          }
        }
      }
      event Value Change {
        n154 = event-data() -> ()  [unwired: 1 in, 4 out]
        n155 = case shown="True" "?" {
          tunnel: w284 -> [w286 w291]
          frame False {
            w288 = T2 11 items=["PXI_TRIG0", "PXI_TRIG1", "PXI_TRIG2", "PXI_TRIG3", "PXI_TRIG4", "PXI_TRIG5", "PXI_TRIG6", "PXI_TRIG7", "PXIE_DSTARA", "PXIE_DSTARB", "PXI_STAR", "PXIE_DSTARC"] ("pxi signal")
            # "Disable PXI Signal"
            n156 = call <instrlib>:"Write PXI Signal.vi"("signal value"=FALSE, "pxi signal"=w288, "core handle in"=w286) -> ()  [unwired: 7 in, 2 out]
          }
          frame True {
            w290 = T2 11 items=["PXI_TRIG0", "PXI_TRIG1", "PXI_TRIG2", "PXI_TRIG3", "PXI_TRIG4", "PXI_TRIG5", "PXI_TRIG6", "PXI_TRIG7", "PXIE_DSTARA", "PXIE_DSTARB", "PXI_STAR", "PXIE_DSTARC"] ("pxi signal")
            # "Enable PXI Signal"
            n157 = call <instrlib>:"Write PXI Signal.vi"("signal value"=TRUE, "pxi signal"=w290, "core handle in"=w291) -> ()  [unwired: 7 in, 2 out]
          }
        }
      }
    }
  }
  n158 = call <instrlib>:"Close.vi"("error in (no error)"=w15, "core handle in"=w14) -> ()  [unwired: 8 in, 2 out]
